vi "TcA02-008_MutualExclusionWhenModifyingAttributes.vi"(1 "Input buffer":T3="1", 3 "Invocation info":T2, 5 "error in (no error)":errorcluster, 6 "Add log to result?":bool) -> (16 "Test Data":T1 {"Numeric Measurement" format="%.2f"}, 19 "error out":errorcluster)   [LabVIEW 2009]
doc: "Test case template."
uses:
  Shared/Support_InputBuffer.ctl
  Shared/Support_InvocationInfo.ctl
  Shared/Support_TestData.ctl
  TestClasses/G#BaseClass1_class/G#BaseClass1.lvclass
  TestClasses/G#SubClass2_class/G#SubClass2.lvclass
  TestClasses/G#BaseClass2_class/G#BaseClass2.lvclass
  <vilib>/addons/_AddQ/G#Object/G#Object.lvclass
panel:
  in  "Test name":string="TcA02-008 Mutual exclusion when modifying attributes"
  out "Test result":bool
  out "Result":string
  # "Verify that objects attributes can be modified exclusively and any\nthat tries to modify the attributes will be mutual excluded and forced\nto wait until attributes are unlocked again."
  # "Sub test case"
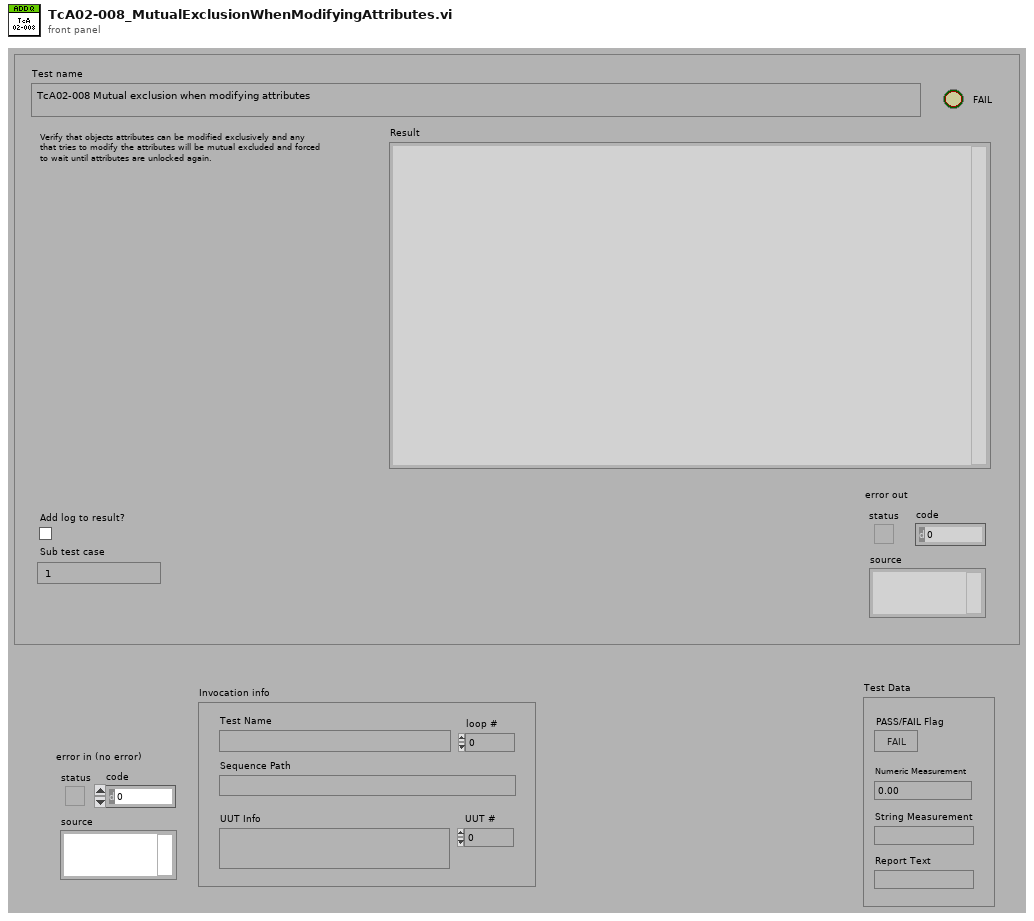
[diagram p1: front panel]
types:
  T1 = typedef "Support_TestData.ctl" = cluster{"PASS/FAIL Flag":bool, "Numeric Measurement":dbl, "String Measurement":string, "Report Text":string}
  T2 = typedef "Support_InvocationInfo.ctl" = cluster{"UUT #":i32, "loop #":i32, "UUT Info":string, "Test Name":string, "Sequence Path":path}
  T3 = typedef "Support_InputBuffer.ctl" = string
  T4 = typedef "Support_ResultType.ctl" = cluster{"Pass":bool, "Comment":string, "MeasurementValue":dbl}
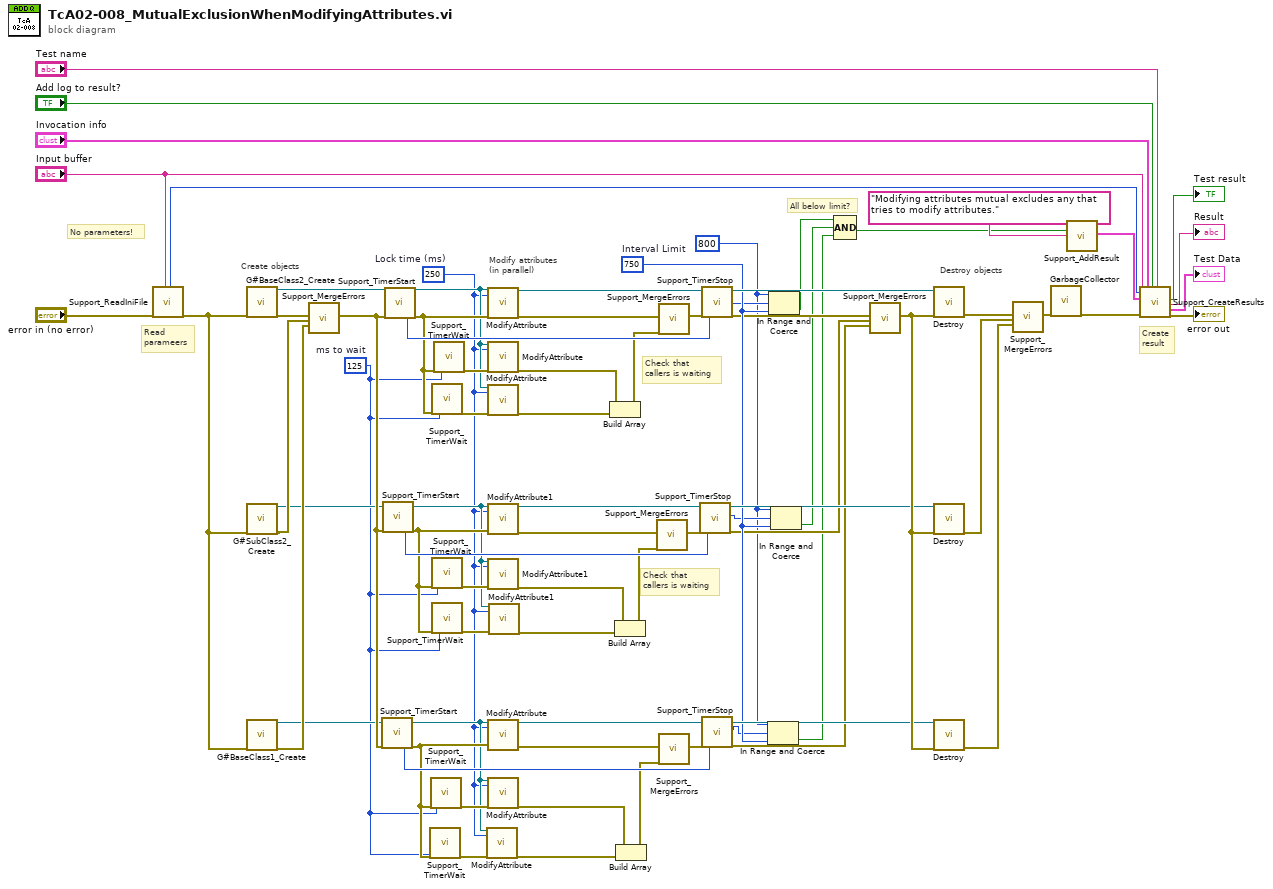
[diagram p0: block diagram]
diagram:
  w3 = u32 800 ("upper limit")
  w33 = u32 750  # Interval Limit
  w11 = u32 250  # Lock time (ms)
  w10 = u32 125  # ms to wait
  # "Check that\ncallers is waiting"
  # "Check that\ncallers is waiting"
  # "All below limit?"
  # "Destroy objects"
  # "Modify attributes\n(in parallel)"
  # "Create objects"
  # "No parameters!"
  # "Create\nresult"
  # "Read\nparameers"
  n1 = call "Support_ReadIniFile.vi"("error in (no error)"="error in (no error)", "Sub test case"="Input buffer") -> ("Timer start"=w61:u32, "error out"=w56:errorcluster)  [unwired: 10 in, 6 out]
  n2 = call "G#BaseClass2_Create.vi"("error in (no error)"=w56) -> ("reference out"=w29:refnum<class "G#BaseClass2.lvclass">, "error out"=w39:errorcluster)  [unwired: 17 in]
  n3 = call "G#SubClass2_Create.vi"("error in (no error)"=w56) -> ("reference out"=w16:refnum<class "G#SubClass2.lvclass">, "error out"=w38:errorcluster)  [unwired: 17 in]
  n4 = call "G#BaseClass1_Create.vi"("error in (no error)"=w56) -> ("reference out"=w12:refnum<class "G#BaseClass1.lvclass">, "error out"=w37:errorcluster)  [unwired: 16 in, 1 out]
  n5 = call "Support_MergeErrors.vi"("error in 1"=w39, "error in 2"=w38, "error in 3"=w37) -> ("error out"=w52:errorcluster)  [unwired: 15 in, 1 out]
  n6 = call "Support_TimerStart.vi"("error in (no error)"=w52) -> ("Start time"=w46:u32, "error out"=w14:errorcluster)  [unwired: 17 in]
  n7 = call "Support_TimerStart.vi"("error in (no error)"=w52) -> ("Start time"=w47:u32, "error out"=w20:errorcluster)  [unwired: 17 in]
  n8 = call "Support_TimerStart.vi"("error in (no error)"=w52) -> ("Start time"=w53:u32, "error out"=w30:errorcluster)  [unwired: 17 in]
  n9 = call "Support_TimerWait.vi"("error in (no error)"=w14, "milliseconds to wait"=w10) -> ("error out"=w13:errorcluster)  [unwired: 17 in]
  n10 = call "Support_TimerWait.vi"("error in (no error)"=w14, "milliseconds to wait"=w10) -> ("error out"=w15:errorcluster)  [unwired: 17 in]
  n11 = call "Support_TimerWait.vi"("error in (no error)"=w30, "milliseconds to wait"=w10) -> ("error out"=w31:errorcluster)  [unwired: 17 in]
  n12 = call "Support_TimerWait.vi"("error in (no error)"=w20, "milliseconds to wait"=w10) -> ("error out"=w22:errorcluster)  [unwired: 17 in]
  n13 = call "Support_TimerWait.vi"("error in (no error)"=w20, "milliseconds to wait"=w10) -> ("error out"=w21:errorcluster)  [unwired: 17 in]
  n14 = call "Support_TimerWait.vi"("error in (no error)"=w30, "milliseconds to wait"=w10) -> ("error out"=w32:errorcluster)  [unwired: 17 in]
  n15 = call-dynamic "ModifyAttribute.vi"("reference in"=w12, "Lock time (ms)"=w11, "error in (no error)"=w13) -> ("error out"=w9:errorcluster)  [unwired: 15 in, 1 out]
  n16 = call-dynamic "ModifyAttribute.vi"("reference in"=w29, "Lock time (ms)"=w11, "error in (no error)"=w30) -> ("reference out"=w44:refnum<class "G#BaseClass2.lvclass">, "error out"=w55:errorcluster)  [unwired: 14 in, 1 out]
  n17 = call-dynamic "ModifyAttribute.vi"("reference in"=w29, "Lock time (ms)"=w11, "error in (no error)"=w32) -> ("error out"=w25:errorcluster)  [unwired: 14 in, 2 out]
  n18 = call-dynamic "ModifyAttribute.vi"("reference in"=w29, "Lock time (ms)"=w11, "error in (no error)"=w31) -> ("error out"=w24:errorcluster)  [unwired: 14 in, 2 out]
  n19 = call-dynamic "ModifyAttribute1.vi"("reference in"=w16, "Lock time (ms)"=w11, "error in (no error)"=w20) -> ("reference out"=w43:refnum<class "G#SubClass2.lvclass">, "error out"=w49:errorcluster)  [unwired: 14 in, 1 out]
  n20 = call-dynamic "ModifyAttribute1.vi"("reference in"=w16, "Lock time (ms)"=w11, "error in (no error)"=w22) -> ("error out"=w17:errorcluster)  [unwired: 14 in, 2 out]
  n21 = call-dynamic "ModifyAttribute.vi"("reference in"=w12, "Lock time (ms)"=w11, "error in (no error)"=w14) -> ("reference out"=w42:refnum<class "G#BaseClass1.lvclass">, "error out"=w51:errorcluster)  [unwired: 15 in]
  n22 = call-dynamic "ModifyAttribute.vi"("reference in"=w12, "Lock time (ms)"=w11, "error in (no error)"=w15) -> ("error out"=w8:errorcluster)  [unwired: 15 in, 1 out]
  n23 = call-dynamic "ModifyAttribute1.vi"("reference in"=w16, "Lock time (ms)"=w11, "error in (no error)"=w21) -> ("error out"=w19:errorcluster)  [unwired: 14 in, 2 out]
  n24 = Build Array(w25, w24) -> (w23:errorcluster[])
  n25 = Build Array(w17, w19) -> (w18:errorcluster[])
  n26 = Build Array(w8, w9) -> (w7:errorcluster[])
  n27 = call "Support_MergeErrors.vi"("error in 1"=w49, "Error array"=w18) -> ("error out"=w48:errorcluster)  [unwired: 16 in, 1 out]
  n28 = call "Support_MergeErrors.vi"("error in 1"=w55, "Error array"=w23) -> ("error out"=w54:errorcluster)  [unwired: 16 in, 1 out]
  n29 = call "Support_MergeErrors.vi"("error in 1"=w51, "Error array"=w7) -> ("error out"=w50:errorcluster)  [unwired: 16 in, 1 out]
  n30 = call "Support_TimerStop.vi"("error in (no error)"=w48, "Start time"=w47) -> ("Time (ms)"=w5:u32, "error out"=w27:errorcluster)  [unwired: 16 in]
  n31 = call "Support_TimerStop.vi"("error in (no error)"=w54, "Start time"=w53) -> ("Time (ms)"=w6:u32, "error out"=w28:errorcluster)  [unwired: 16 in]
  n32 = call "Support_TimerStop.vi"("error in (no error)"=w50, "Start time"=w46) -> ("Time (ms)"=w4:u32, "error out"=w26:errorcluster)  [unwired: 16 in]
  n33 = In Range and Coerce(upper limit=w3, x=w4, lower limit=w33) -> (In Range?=w1:bool)  [unwired: 1 out]
  n34 = In Range and Coerce(upper limit=w3, x=w6, lower limit=w33) -> (In Range?=w41:bool)  [unwired: 1 out]
  n35 = In Range and Coerce(upper limit=w3, x=w5, lower limit=w33) -> (In Range?=w2:bool)  [unwired: 1 out]
  n36 = Compound Arithmetic op=AND(w41, w2, w1) -> (w40:bool)
  n37 = call "Support_MergeErrors.vi"("error in 1"=w28, "error in 2"=w27, "error in 3"=w26) -> ("error out"=w45:errorcluster)  [unwired: 15 in, 1 out]
  n38 = call-dynamic "Destroy.vi"("reference in"=w44, "error in (no error)"=w45) -> ("error out"=w36:errorcluster)  [unwired: 16 in, 1 out]
  n39 = call-dynamic "Destroy.vi"("reference in"=w43, "error in (no error)"=w45) -> ("error out"=w35:errorcluster)  [unwired: 16 in, 1 out]
  n40 = call-dynamic "Destroy.vi"("reference in"=w42, "error in (no error)"=w45) -> ("error out"=w34:errorcluster)  [unwired: 16 in, 1 out]
  n41 = call "Support_MergeErrors.vi"("error in 1"=w36, "error in 2"=w35, "error in 3"=w34) -> ("error out"=w60:errorcluster)  [unwired: 15 in, 1 out]
  n42 = call <vilib>:"GarbageCollector.vi"("error in (no error)"=w60) -> ("error out"=w59:errorcluster)  [unwired: 16 in, 2 out]
  n43 = call "Support_AddResult.vi"("Pass"=w40, "Comment"="Modifying attributes mutual excludes any that tries to modify attributes.") -> ("Results out"=w58:T4[])  [unwired: 17 in]
  n44 = call "Support_CreateResults.vi"("Sub test case"="Input buffer", "Timer start"=w61, "Results"=w58, "error in (no error)"=w59, "Invocation info"="Invocation info", "Add log to result?"="Add log to result?", "Test name"="Test name") -> ("Pass/fail flag"=→"Test result":bool, "Result"=→"Result":string, "Test Data"=→"Test Data":T1, "error out"=→"error out":errorcluster)  [unwired: 9 in]
